vi "escalon_lab1.vi"() -> ()   [LabVIEW 2025]
uses:
  <vilib>/Utility/file.llb/Write Delimited Spreadsheet (DBL).vi
panel:
  in  "Voltaje":dbl
  out "Waveform Chart":dynamicdata(graph)
  out "Rpm":dbl
  in  "stop (F)":bool
  # "Voltaje [V]"
  # "Velocidad [RPM]"
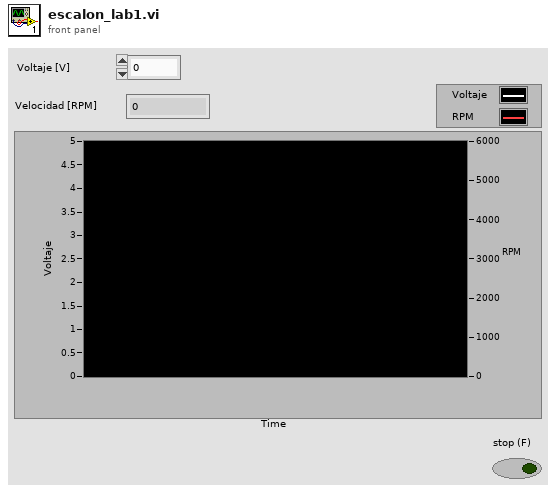
[diagram p1: front panel]
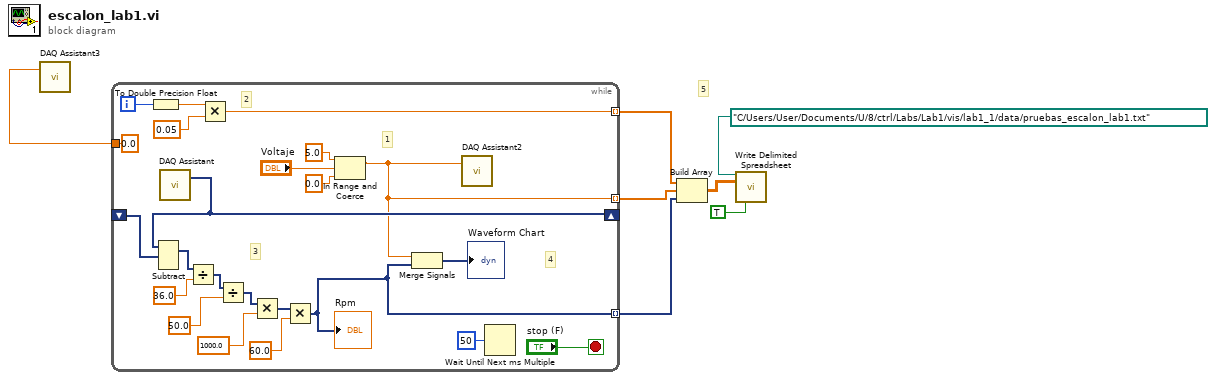
[diagram p0: block diagram]
diagram:
  # "5"
  n1 = while {
    shift-right: [w28] -> _
    shift-left: _ -> [w27]
    tunnel: [0.0 ("data")] -> w7
    tunnel: [w11] -> w6 mode=indexing
    tunnel: [w16] -> w5 mode=indexing
    tunnel: [w12] -> w4 mode=indexing
    i -> [w15]
    stop <- "stop (F)" stop-if-true
    # "4"
    # "3"
    # "2"
    # "1"
    n2 = To Double Precision Float(number=w15) -> (double precision float=w14:dbl)
    n3 = call "DAQ Assistant"() -> ("data"=w28:dynamicdata)  [unwired: 16 in, 3 out]
    n4 = Subtract(1:w27, 2:w28) -> (0:w20:dynamicdata)  [unwired: 1 in, 1 out]
    n5 = Divide(x=w20, y=36.0) -> (x/y=w18:dynamicdata)
    n6 = Multiply(x=w14, y=0.05) -> (x*y=w12:dbl)
    n7 = Divide(x=w18, y=50.0) -> (x/y=w19:dynamicdata)
    n8 = Multiply(x=w19, y=1000.0) -> (x*y=w25:dynamicdata)
    n9 = Multiply(x=w25, y=60.0) -> (x*y=w16:dynamicdata)
    "Rpm" <- w16
    n10 = In Range and Coerce(upper limit=5.0, x="Voltaje", lower limit=0.0) -> (coerced(x)=w11:dbl)  [unwired: 1 out]
    n11 = Merge Signals(w11, w16) -> (→"Waveform Chart":dynamicdata)
    n12 = call "DAQ Assistant2"("data"=w11) -> ()  [unwired: 17 in, 2 out]
    n13 = Wait Until Next ms Multiple(millisecond multiple=u32 50) -> ()  [unwired: 1 out]
  }
  n14 = call "DAQ Assistant3"("data"=w7) -> ()  [unwired: 17 in, 2 out]
  n15 = Build Array(w4, w6, w5) -> (w2:dbl[][])
  n16 = call-poly <vilib>:"Write Delimited Spreadsheet.vi"("file path (dialog if empty)"=path "C:/Users/User/Documents/U/8/ctrl/Labs/Lab1/vis/lab1_1/data/pruebas_escalon_lab1.txt", "2D data"=w2, "transpose? (no:F)"=TRUE) -> ()  [unwired: 11 in, 2 out]
